vi "Search 1D String Array First Match.vi"(1 "Start index (0)":i32, 2 "Element":string, 3 "1D String Array":string[](array[string])) -> (0 "Index":i32)   [LabVIEW 2014, in "SLL String.lvlib"]
doc: "Search 1D String Array for a specified element ignoring white space and case sensitivity"
uses:
  SLL String.lvlib
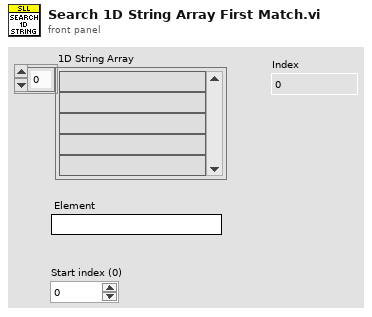
[diagram p1: front panel]
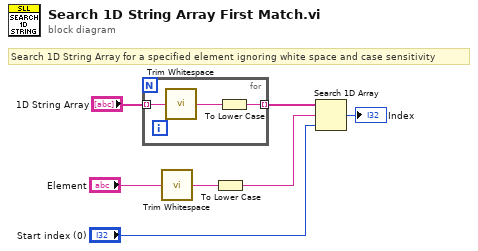
[diagram p0: block diagram]
diagram:
  # "Search 1D String Array for a specified element ignoring white space and case sensitivity"
  n1 = for {
    tunnel: "1D String Array" -> [w10] mode=indexing
    tunnel: [w8] -> w3 mode=indexing
    n2 = call <vilib>:"Trim Whitespace.vi"("string"=w10) -> ("trimmed string"=w9:string)  [unwired: 1 in]
    n3 = To Lower Case(string=w9) -> (all lower case string=w8:string)
  }
  n4 = call <vilib>:"Trim Whitespace.vi"("string"="Element") -> ("trimmed string"=w5:string)  [unwired: 1 in]
  n5 = To Lower Case(string=w5) -> (all lower case string=w2:string)
  n6 = Search 1D Array(1D array=w3, element=w2, start index (0)="Start index (0)") -> (index of element=→"Index":i32)
